vi "Matches.vi"(8 "error in (no error)":errorcluster, 10 "Actual":variant, 11 "IsFalse in":refnum<class "IsFalse.lvclass">) -> (0 "error out":errorcluster, 2 "Result":bool, 3 "IsFalse out":refnum<class "IsFalse.lvclass">)   [LabVIEW 2017, in "Transparent Assertions.lvlib" / "IsFalse.lvclass"]
doc: "Evaluates the constraint for <B>Actual</B>. Returns true if the constraint is met."
uses:
  IsFalse.lvclass
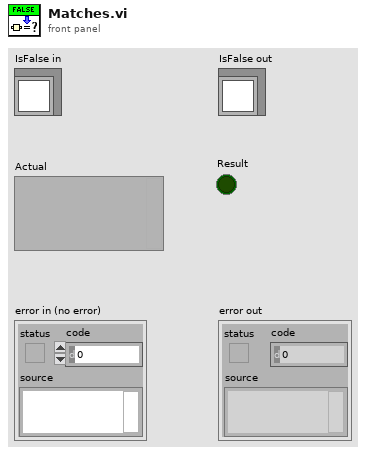
[diagram p1: front panel]
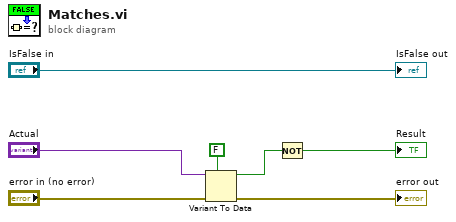
[diagram p0: block diagram]
diagram:
  n1 = Variant To Data(error in="error in (no error)", type=FALSE, Variant="Actual") -> (data=w1:bool, error out=→"error out":errorcluster)
  n2 = Not(x=w1) -> (.not. x?=→"Result":bool)
  "IsFalse out" <- "IsFalse in"
